vi "Read_ASCII.vi"(6 "Number of Columns":i32=8, 9 "Prompt":string="Please select ASCII\nOPTOPTRAK file") -> (0 "Output":sgl[][](array[numeric]) format="%.5f")   [LabVIEW 2016]
panel:
  # "OPTOTRAK"
  # "This program reads ASCII files prduced by \nOPTOTRAK DAP FL_ASCII\n\nBy Americo A Migliaccio         20 Oct 98"
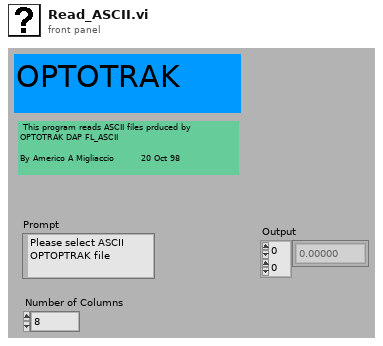
[diagram p1: front panel]
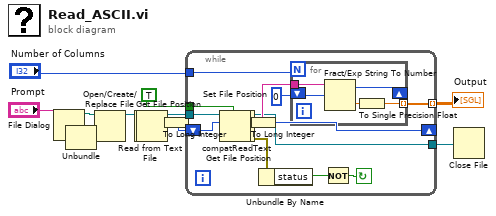
[diagram p0: block diagram]
diagram:
  n1 = File Dialog(7:"Prompt") -> (0:w4:errorcluster, 3:w13:path)  [unwired: 6 in, 2 out]
  n2 = Unbundle(w4) -> ()  [unwired: 3 out]
  n3 = Open/Create/Replace File(file path (use dialog)=w13) -> (refnum out=w12:refnum<file>)  [unwired: 5 in, 2 out]
  n4 = Read from Text File(file (use dialog)=w12) -> (refnum out=w3:refnum<file>, error out=w2:errorcluster)  [unwired: 3 in, 2 out]
  n5 = Get File Position(4:w2, 7:w3) -> (2:w1:i64, 3:w9:refnum<file>)  [unwired: 1 out]
  n6 = To Long Integer(number=w1) -> (32bit integer=w11:i32)
  n7 = while {
    tunnel: "Number of Columns" -> [w19]
    tunnel: [w20] -> w7
    tunnel: [w21] -> w8 mode=indexing
    tunnel: w9 -> [w28]
    tunnel: TRUE ("line mode (F)") -> [w29]
    shift-left: w11 -> [w30]
    shift-right: [w27] -> _
    stop <- w24 continue-if-true
    n8 = Set File Position(offset (in bytes) (0)=w30, refnum=w28) -> (refnum out=w18:refnum<file>, error out=w17:errorcluster)  [unwired: 2 in]
    n9 = call <vilib>:"compatReadText.vi"("line mode (F)"=w29, "error in"=w17, "refnum"=w18) -> ("error out"=w15:errorcluster, "data"=w23:string, "dup refnum"=w16:refnum<file>)  [unwired: 6 in]
    n10 = Get File Position(4:w15, 7:w16) -> (0:w26:errorcluster, 2:w14:i64, 3:w20:refnum<file>)
    n11 = To Long Integer(number=w14) -> (32bit integer=w27:i32)
    n12 = Unbundle By Name(w26) -> ("status"=w25:bool)
    n13 = for {
      N: w19 -> [_]
      tunnel: w23 -> [w35]
      shift-right: [w33] -> _
      shift-left: 0 ("offset past number") -> [w34]
      tunnel: [w31] -> w21 mode=indexing
      n14 = Fract/Exp String To Number(string=w35, offset=w34) -> (offset past number=w33:i32, number=w32:dbl)  [unwired: 2 in]
      n15 = To Single Precision Float(number=w32) -> (single precision float=w31:sgl)
    }
    n16 = Not(x=w25) -> (.not. x?=w24:bool)
  }
  "Output" <- w8
  n17 = Close File(refnum=w7) -> ()  [unwired: 1 in, 2 out]
